vi "PIDs.vi"(8 "error in (no error)":errorcluster, 11 "Node Ptr":T1 format="%.0x") -> (0 "error out":errorcluster)   [LabVIEW 2015, in "Diagnostics Addon System Explorer.lvlib"]
uses:
  Diagnostics Addon System Explorer.lvlib
  <vilib>/NI Veristand/Custom Device API/Custom Device Item Ref.ctl
  Shared/FG Action.ctl
  Shared/GUID Lookup.vi
  <vilib>/NI Veristand/Custom Device API/NI VeriStand - Set Item Property.vi
  <vilib>/NI Veristand/Custom Device API/Set Item Property (U32).vi
  <vilib>/NI Veristand/Custom Device API/NI VeriStand - Get Item Property.vi
  <vilib>/NI Veristand/Custom Device API/Get Item Property (U32).vi
  <vilib>/NI Veristand/Custom Device API/Custom Device API.lvlib
  Shared/Diagnostics Addon Shared.lvlib
panel:
  in  "Description":string
  in  "SHDocVw.IWebBrowser":refnum<k7>(container)
  out "PIDs":i32(listbox)
  out "Name":string
  in  "Header":cluster{"Section Name":string}={"Section Name"="Custom Device Item Settings"}
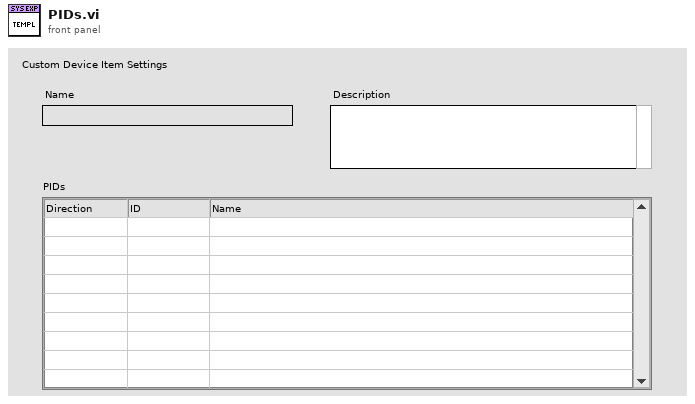
[diagram p1: front panel]
types:
  T1 = typedef "Custom Device API.lvlib/Custom Device Item Ref.ctl" = u64
  T2 = typedef "Diagnostics Addon Shared.lvlib/FG Action.ctl" = enum16{"Get", "Set"}
  T3 = typedef "Custom Device API.lvlib/Custom Device Item Info.ctl" = cluster{"Name":string, "Is Channel":bool, "GUID":string, "Is Waveform":bool}
  T4 = typedef "Custom Device API.lvlib/Custom Device Commands.ctl" = enum16{"Default", "Item renamed", "Shutdown", "Dynamic button pressed"}
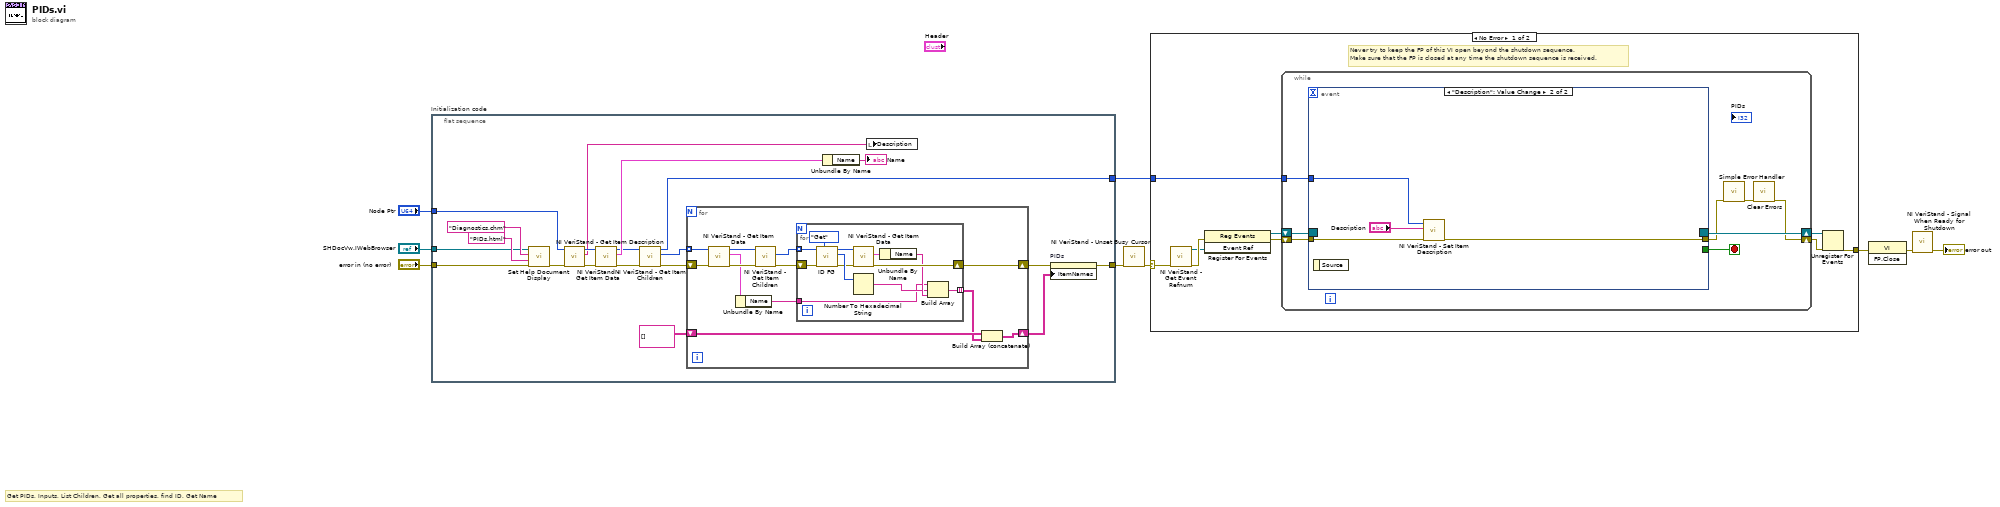
[diagram p0: block diagram]
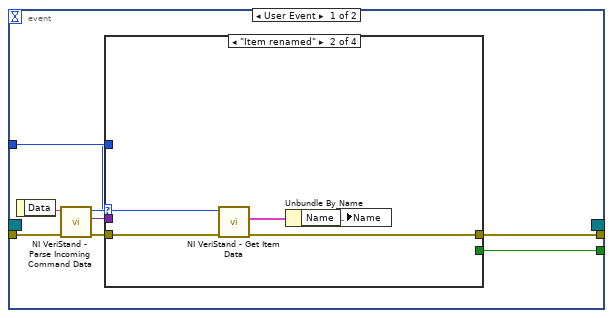
[diagram p2: hidden frame]
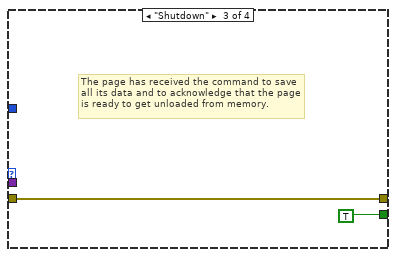
[diagram p4: hidden frame]
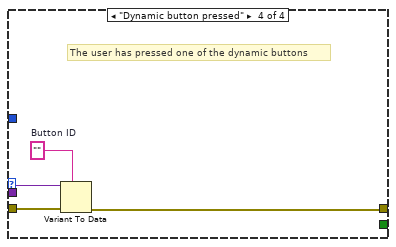
[diagram p5: hidden frame]
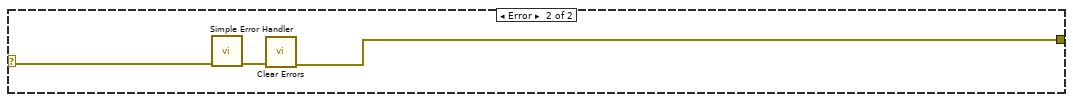
[diagram p6: hidden frame]
diagram:
  # "Get PIDs, Inputs, List Children, Get all properties, find ID, Get Name"
  n1 = flat-sequence "Initialization code" {
    tunnel: "error in (no error)" -> [w23]
    tunnel: "Node Ptr" -> [w28]
    tunnel: [w19] -> w5
    tunnel: [w15] -> w2
    tunnel: "SHDocVw.IWebBrowser" -> [w21]
    frame #0 {
      n2 = call "Set Help Document Display.vi"("error in (no error)"=w23, "HTML File"="PIDs.html", "Main CHM File"="Diagnostics.chm", "SHDocVw.IWebBrowser2"=w21) -> ("error out"=w22:errorcluster)  [unwired: 7 in]
      n3 = call <vilib>:"NI VeriStand - Get Item Description.vi"("error in (no error)"=w22, "Item Ref in"=w28) -> ("error out"=w27:errorcluster, "Description"=w10:string, "Item Ref out"=w29:T1)  [unwired: 7 out]
      n4 = call <vilib>:"NI VeriStand - Get Item Data.vi"("error in (no error)"=w27, "Item Ref in"=w29) -> ("error out"=w18:errorcluster, "Item Info"=w26:T3, "Item Ref out"=w17:T1)  [unwired: 7 out]
      n5 = call <vilib>:"NI VeriStand - Get Item Children.vi"("error in (no error)"=w18, "Item Ref in"=w17) -> ("error out"=w16:errorcluster, "Child Refs"=w14:T1[], "Item Ref out"=w15:T1)  [unwired: 6 in, 1 out]
      n6 = for {
        tunnel: w14 -> [w33] mode=indexing
        shift-right: [w41] -> w20
        shift-left: w16 -> [w38]
        shift-right: [w30] -> w12
        shift-left: string[][] [] -> [w32]
        n7 = call <vilib>:"NI VeriStand - Get Item Data.vi"("error in (no error)"=w38, "Item Ref in"=w33) -> ("error out"=w37:errorcluster, "Item Info"=w35:T3, "Item Ref out"=w36:T1)  [unwired: 7 out]
        n8 = Unbundle By Name(w35) -> ("Name"=w34:string)
        n9 = call <vilib>:"NI VeriStand - Get Item Children.vi"("error in (no error)"=w37, "Item Ref in"=w36) -> ("error out"=w39:errorcluster, "Child Refs"=w40:T1[])  [unwired: 6 in, 2 out]
        n10 = for {
          tunnel: w40 -> [w53] mode=indexing
          shift-right: [w49] -> w41
          shift-left: w39 -> [w52]
          tunnel: [w44] -> w31 mode=indexing
          tunnel: w34 -> [w43]
          n11 = call "ID FG.vi"("Action"=FG_Action."Get", "error in (no error)"=w52, "Device Item Ref in"=w53) -> ("error out"=w50:errorcluster, "ID"=w51:u32, "Device Item Ref out"=w48:T1)  [unwired: 6 in]
          n12 = call <vilib>:"NI VeriStand - Get Item Data.vi"("error in (no error)"=w50, "Item Ref in"=w48) -> ("error out"=w49:errorcluster, "Item Info"=w47:T3)  [unwired: 8 out]
          n13 = Number To Hexadecimal String(2:w51) -> (0:w45:string)  [unwired: 1 in]
          n14 = Unbundle By Name(w47) -> ("Name"=w46:string)
          n15 = Build Array(w43, w45, w46) -> (w44:string[])
        }
        n16 = Build Array (concatenate)(w32, w31) -> (w30:string[][])
      }
      n17 = Unbundle By Name(w26) -> ("Name"=→"Name":string)
      n18 = local write "Description"(w10) -> ()
      n19 = property on="PIDs" class="MCListbox (strict)"(error in=w20, "ItemNames"=w12) -> (error out=w19:errorcluster)  [unwired: 1 in, 1 out]
    }
  }
  n20 = call <vilib>:"NI VeriStand - Unset Busy Cursor.vi"("error in (no error)"=w5) -> ("error out"=w4:errorcluster)  [unwired: 10 out]
  n21 = case shown="No Error" w4 {
    selector: w4 -> [w54 w97]
    tunnel: [w59 w95] -> w9
    tunnel: w2 -> [w55 _]
    frame No Error {
      # "Never try to keep the FP of this VI open beyond the shutdown sequence.\nMake sure that the FP is closed at any time the shutdown sequence is received."
      n22 = call <vilib>:"NI VeriStand - Get Event Refnum.vi"("error in (no error)"=w54) -> ("error out"=w62:errorcluster, "Event Ref"=w58:refnum<user-event>)  [unwired: 9 out]
      n23 = register-events(error in=w62, w58) -> (reference out=w56:refnum<event-registration>, error out=w57:errorcluster)  [unwired: 1 in]
      n24 = while {
        tunnel: w55 -> [w66]
        shift-right: [w63] -> w60
        shift-left: w57 -> [w69]
        shift-right: [w70] -> w61
        shift-left: w56 -> [w68]
        stop <- w67 stop-if-true
        n25 = event shown="[1] \"Description\": Value Change" {
          selector: w68 -> [_ _]
          dyn-events: [_ _] -> w70
          timeout: _ -> [_ _]
          tunnel: w69 -> [w78 w93]
          tunnel: [w74 _] -> w67
          tunnel: [w73 w91] -> w65
          tunnel: w66 -> [w72 w94]
          event User Event {
            n26 = event-data() -> ("Data"=w77:string)  [unwired: 1 out]
            n27 = call <vilib>:"NI VeriStand - Parse Incoming Command Data.vi"("error in (no error)"=w78, "Incoming data"=w77) -> ("error out"=w76:errorcluster, "Outgoing data"=w71:variant, "Action"=w75:T4)  [unwired: 7 out]
            n28 = case shown="\"Item renamed\"" w75 {
              tunnel: w76 -> [w79 w84 w85 w90]
              tunnel: [_ _ TRUE _] -> w74
              tunnel: [w79 w81 w85 w87] -> w73
              tunnel: w72 -> [_ w83 _ _]
              tunnel: w71 -> [_ _ _ w89]
              frame "Default", Default {
              }
              frame "Item renamed" {
                n29 = call <vilib>:"NI VeriStand - Get Item Data.vi"("error in (no error)"=w84, "Item Ref in"=w83) -> ("error out"=w81:errorcluster, "Item Info"=w82:T3)  [unwired: 8 out]
                n30 = Unbundle By Name(w82) -> ("Name"=w80:string)
                n31 = local write "Name"(w80) -> ()
              }
              frame "Shutdown" {
                # "The page has received the command to save all its data and to acknowledge that the page is ready to get unloaded from memory."
              }
              frame "Dynamic button pressed" {
                w88 = ""  # Button ID
                # "The user has pressed one of the dynamic buttons"
                n32 = Variant To Data(error in=w90, type=w88, Variant=w89) -> (error out=w87:errorcluster)  [unwired: 1 out]
              }
            }
          }
          event "Description": Value Change {
            n33 = event-data() -> ()  [unwired: 2 out]
            n34 = call <vilib>:"NI VeriStand - Set Item Description.vi"("error in (no error)"=w93, "Description"="Description", "Item Ref in"=w94) -> ("error out"=w91:errorcluster)  [unwired: 8 out]
          }
        }
        n35 = call <vilib>:"Simple Error Handler.vi"("error in (no error)"=w65) -> ("error out"=w64:errorcluster)  [unwired: 1 in, 7 out]
        n36 = call <vilib>:"Clear Errors.vi"("error in (no error)"=w64) -> ("error out"=w63:errorcluster)  [unwired: 1 in, 5 out]
      }
      n37 = Unregister For Events(event registration refnum=w61, error in=w60) -> (error out=w59:errorcluster)
    }
    frame Error {
      n38 = call <vilib>:"Simple Error Handler.vi"("error in (no error)"=w97) -> ("error out"=w96:errorcluster)  [unwired: 1 in, 7 out]
      n39 = call <vilib>:"Clear Errors.vi"("error in (no error)"=w96) -> ("error out"=w95:errorcluster)  [unwired: 1 in, 5 out]
    }
  }
  n40 = invoke class="VI" method="FP.Close"(error in=w9) -> (error out=w8:errorcluster)  [unwired: 2 in, 2 out]
  n41 = call <vilib>:"NI VeriStand - Signal When Ready for Shutdown.vi"("error in (no error)"=w8) -> ("error out"=→"error out":errorcluster)  [unwired: 10 out]
